vi "smartComparison.vi"(6 "whoCares? index":dbl, 9 "Process variable":dbl, 10 "Setpoint":dbl) -> (1 "Happy":bool)   [LabVIEW 2020]
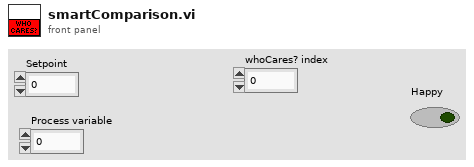
[diagram p1: front panel]
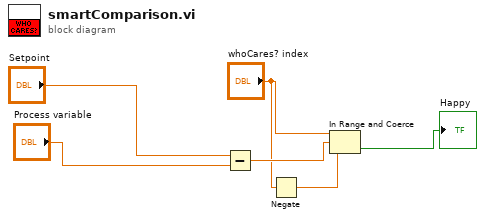
[diagram p0: block diagram]
diagram:
  n1 = Subtract(x="Setpoint", y="Process variable") -> (x-y=w4:dbl)
  n2 = Negate(x="whoCares? index") -> (-x=w3:dbl)
  n3 = In Range and Coerce(upper limit="whoCares? index", x=w4, lower limit=w3) -> (In Range?=→"Happy":bool)  [unwired: 1 out]
